vi "Example3-Race Condition.vi"() -> ()   [LabVIEW 2020]
doc: "This VI demonstate race condition problem."
panel:
  in  "Numeric":i8=10
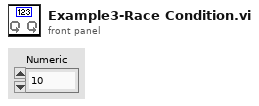
[diagram p1: front panel]
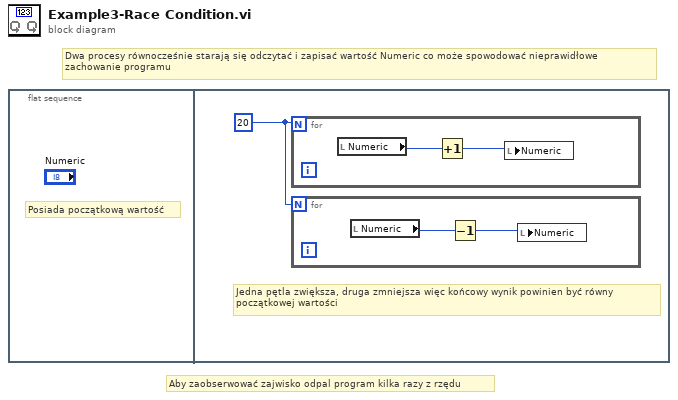
[diagram p0: block diagram]
diagram:
  # "Aby zaobserwować zajwisko odpal program kilka razy z rzędu"
  # "Dwa procesy równocześnie starają się odczytać i zapisać wartość Numeric co może spowodować nieprawidłowe \nzachowanie programu"
  n1 = flat-sequence {
    frame #0 {
      # "Posiada początkową wartość"
    }
    frame #1 {
      w1 = 20
      # "Jedna pętla zwiększa, druga zmniejsza więc końcowy wynik powinien być równy \npoczątkowej wartości"
      n2 = for {
        N: w1 -> [_]
        n3 = local read "Numeric"() -> (w5:i8)
        n4 = Increment(x=w5) -> (x+1=w4:i8)
        n5 = local write "Numeric"(w4) -> ()
      }
      n6 = for {
        N: w1 -> [_]
        n7 = local read "Numeric"() -> (w2:i8)
        n8 = Decrement(x=w2) -> (x-1=w3:i8)
        n9 = local write "Numeric"(w3) -> ()
      }
    }
  }
